vi "Delete Scalar DVR.vi"(8 "error in (no error)":errorcluster, 11 "Scalar DVR in":refnum<data-value>) -> (0 "error out":errorcluster, 3 "Scalar out":refnum<class "Scalar.lvclass">)   [LabVIEW 2013, in "MDSplus.lvlib" / "Scalar.lvclass"]
uses:
  <vilib>/MDSplus/Classes/Data_Class/Scalar_Class/Scalar.lvclass
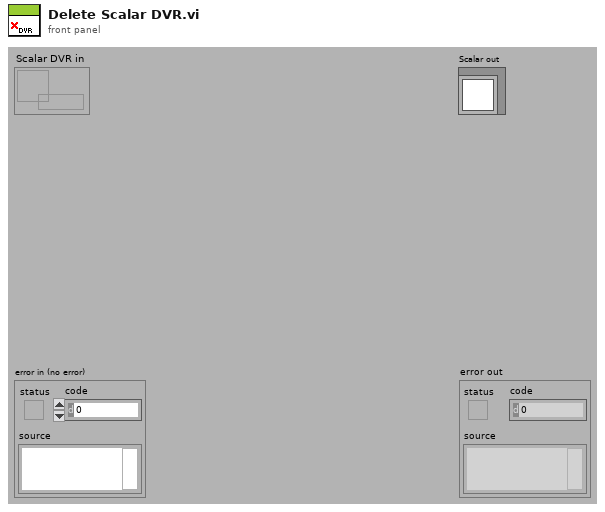
[diagram p1: front panel]
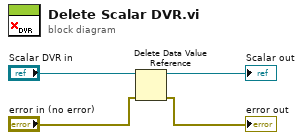
[diagram p0: block diagram]
diagram:
  n1 = Delete Data Value Reference(data value reference="Scalar DVR in", error in="error in (no error)") -> (data value=→"Scalar out":refnum<class "Scalar.lvclass">, error out=→"error out":errorcluster)
